vi "unflattenPlaneAngleFromXML_Scalar.vi"(8 "error in (no error)":errorcluster, 9 "planeAngleUnitInXML":T1, 10 "xmlString":string, 11 "planeAngleForType":dbl[unit]) -> (0 "error out":errorcluster, 3 "planeAngle":dbl[unit])   [LabVIEW 2016, in "UnitsAndXML.lvlib"]
uses:
  <userlib>/Common/UnitsAndXML/UnitsAndXML.lvlib
  <userlib>/Common/UnitsAndXML/FlattenItemWithUnitToXML/FlattenPlaneAngleToXML/PlaneAngleUnit.ctl
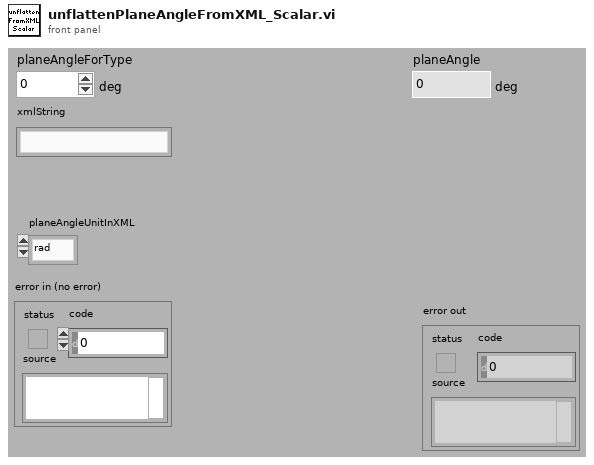
[diagram p1: front panel]
types:
  T1 = typedef "UnitsAndXML.lvlib/PlaneAngleUnit.ctl" = enum16{"rad", "deg", "'", "\""}
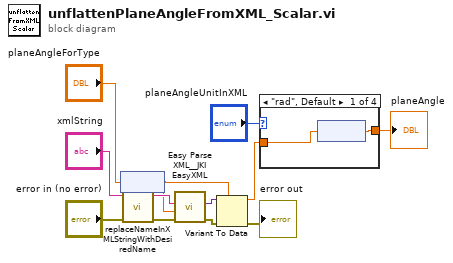
[diagram p0: block diagram]
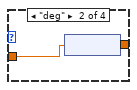
[diagram p2: hidden frame]
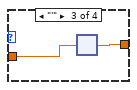
[diagram p3: hidden frame]
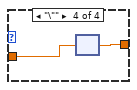
[diagram p4: hidden frame]
diagram:
  n1 = node("planeAngleForType") -> (w7:dbl)
  n2 = call <userlib>:"replaceNameInXMLStringWithDesiredName.vi"("error in"="error in (no error)", "xmlString"="xmlString") -> ("error out"=w1:errorcluster, "revisedXMLString"=w9:string)  [unwired: 8 in]
  n3 = call <vilib>:"Easy Parse XML__JKI EasyXML.vi"("error in (no error)"=w1, "LabVIEW Data (Type)"=w7, "XML String"=w9) -> ("error out"=w4:errorcluster, "LabVIEW Data"=w11:variant)  [unwired: 7 in]
  n4 = Variant To Data(error in=w4, type=w7, Variant=w11) -> (data=w6:dbl, error out=→"error out":errorcluster)
  n5 = case shown="\"rad\", Default" "planeAngleUnitInXML" {
    tunnel: w6 -> [w14 w16 w18 w20]
    tunnel: [w13 w15 w17 w19] -> w5
    frame "rad", Default {
      n6 = node(w14) -> (w13:dbl[unit])
    }
    frame "deg" {
      n7 = node(w16) -> (w15:dbl[unit])
    }
    frame "'" {
      n8 = node(w18) -> (w17:dbl[unit])
    }
    frame "\"" {
      n9 = node(w20) -> (w19:dbl[unit])
    }
  }
  "planeAngle" <- w5
